vi "数据更新.vi"() -> ()   [LabVIEW 2017, in "模块A.lvlib"]
panel:
  out "数值":dbl
  in  "A":dbl=100.0 format="%#_13g"
  out "字符串":string
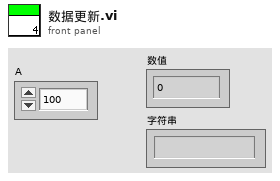
[diagram p1: front panel]
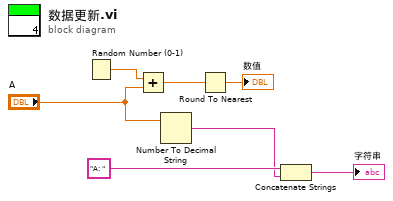
[diagram p0: block diagram]
diagram:
  n1 = Random Number (0-1)() -> (number: 0 to 1=w7:dbl)
  n2 = Add(x=w7, y="A") -> (x+y=w6:dbl)
  n3 = Number To Decimal String(number="A") -> (decimal integer string=w3:string)  [unwired: 1 in]
  n4 = Round To Nearest(number=w6) -> (nearest integer value=→"数值":dbl)
  n5 = Concatenate Strings("A: ", w3) -> (→"字符串":string)
